vi "flatten_cmd_array.vi"(10 "cmd_array":string[](array[string])) -> (2 "cmds":string)   [LabVIEW 2017, in "serial.lvlib"]
uses:
  serial.lvlib
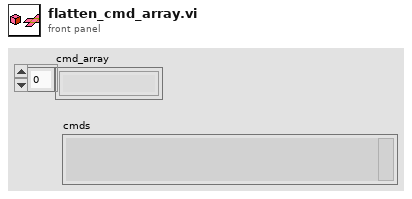
[diagram p1: front panel]
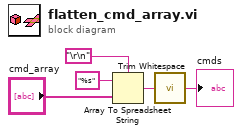
[diagram p0: block diagram]
diagram:
  n1 = Array To Spreadsheet String(delimiter (Tab)="\r\n", array="cmd_array", 3:"%s" ("format string")) -> (spreadsheet string=w3:string)
  n2 = call <vilib>:"Trim Whitespace.vi"("string"=w3) -> ("trimmed string"=→"cmds":string)  [unwired: 1 in]
